vi "Set Mode (uSMC).vi"(8 "error in (no error)":errorcluster, 9 "Index":i32, 11 "Visa Array in":refnum<visa-resource-name>[](array[refnum])) -> (0 "error out":errorcluster, 3 "Visa Array out":refnum<visa-resource-name>[](array[refnum]))   [LabVIEW 2010, in "SignalWriterMH110203USBStepperMotor.lvclass"]
uses:
  SignalWriterMH110203USBStepperMotor.lvclass
  Mode Control (uSMC).ctl
  class_data.vi
panel:
  out "array buffer":u8[](array[numeric]) format="%b"
  out "element":T1={"Turn Buttons Off"=FALSE, "Reduce Current"=TRUE, "Power Off and Make a Whole Step"=TRUE, "Emergency Power Off"=FALSE, "Limit Switch 1 True State"=FALSE, "Limit Switch 2 True State"=FALSE, "Rotary Transducer TRUE State"=TRUE, "Swap Limit Switches"=TRUE, "Limit Switch 1 Operation Enabled"=TRUE, "Limit Switch 2 Operation Enabled"=TRUE, "Rotary Transducer Operation Enabled"=FALSE, "Rotary Transducer Operation Select"=TRUE, "Button 1 True State"=FALSE, "Button 2 True State"=FALSE, "Swap Buttons"=FALSE, "Reset Rotary Transducer Check Positions"=TRUE, "Output Syncronization Enabled"=FALSE, "Reset Output Sync Count"=FALSE, "Sync Operation"=FALSE, "Sync Count"=50, "Power"=TRUE, "Invert Sync Polarity"=FALSE, "Use Encoder"=FALSE, "Invert Encoder Direction"=FALSE, "Reset Encoder To 0"=FALSE, "Reset SM Enc Pos to Enc Pos"=FALSE}
  out "appended array":u8[](array[numeric]) format="%b"
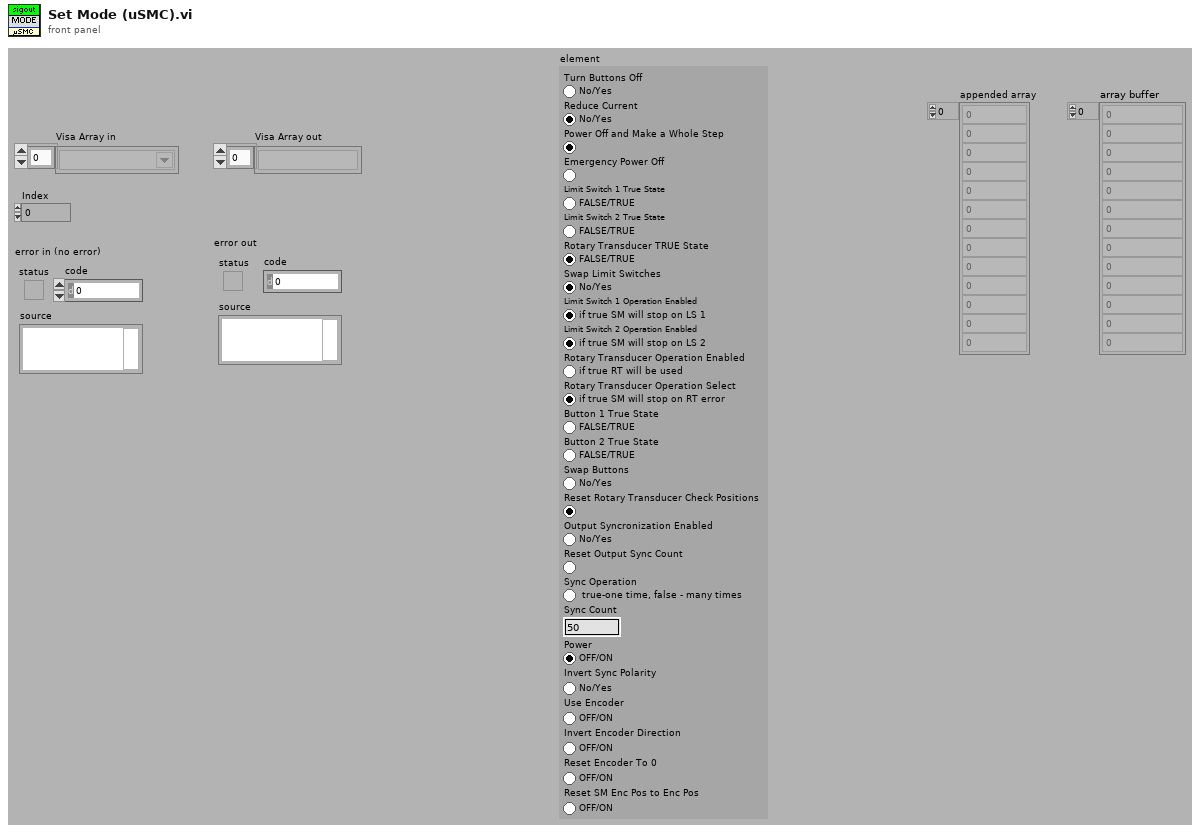
[diagram p1: front panel]
types:
  T1 = typedef "SignalWriterMH110203USBStepperMotor.lvclass/Mode Control (uSMC).ctl" = cluster{"Turn Buttons Off":bool, "Reduce Current":bool, "Power Off and Make a Whole Step":bool, "Emergency Power Off":bool, "Limit Switch 1 True State":bool, "Limit Switch 2 True State":bool, "Rotary Transducer TRUE State":bool, "Swap Limit Switches":bool, "Limit Switch 1 Operation Enabled":bool, "Limit Switch 2 Operation Enabled":bool, "Rotary Transducer Operation Enabled":bool, "Rotary Transducer Operation Select":bool, "Button 1 True State":bool, "Button 2 True State":bool, "Swap Buttons":bool, "Reset Rotary Transducer Check Positions":bool, "Output Syncronization Enabled":bool, "Reset Output Sync Count":bool, "Sync Operation":bool, "Sync Count":u32, "Power":bool, "Invert Sync Polarity":bool, "Use Encoder":bool, "Invert Encoder Direction":bool, "Reset Encoder To 0":bool, "Reset SM Enc Pos to Enc Pos":bool}
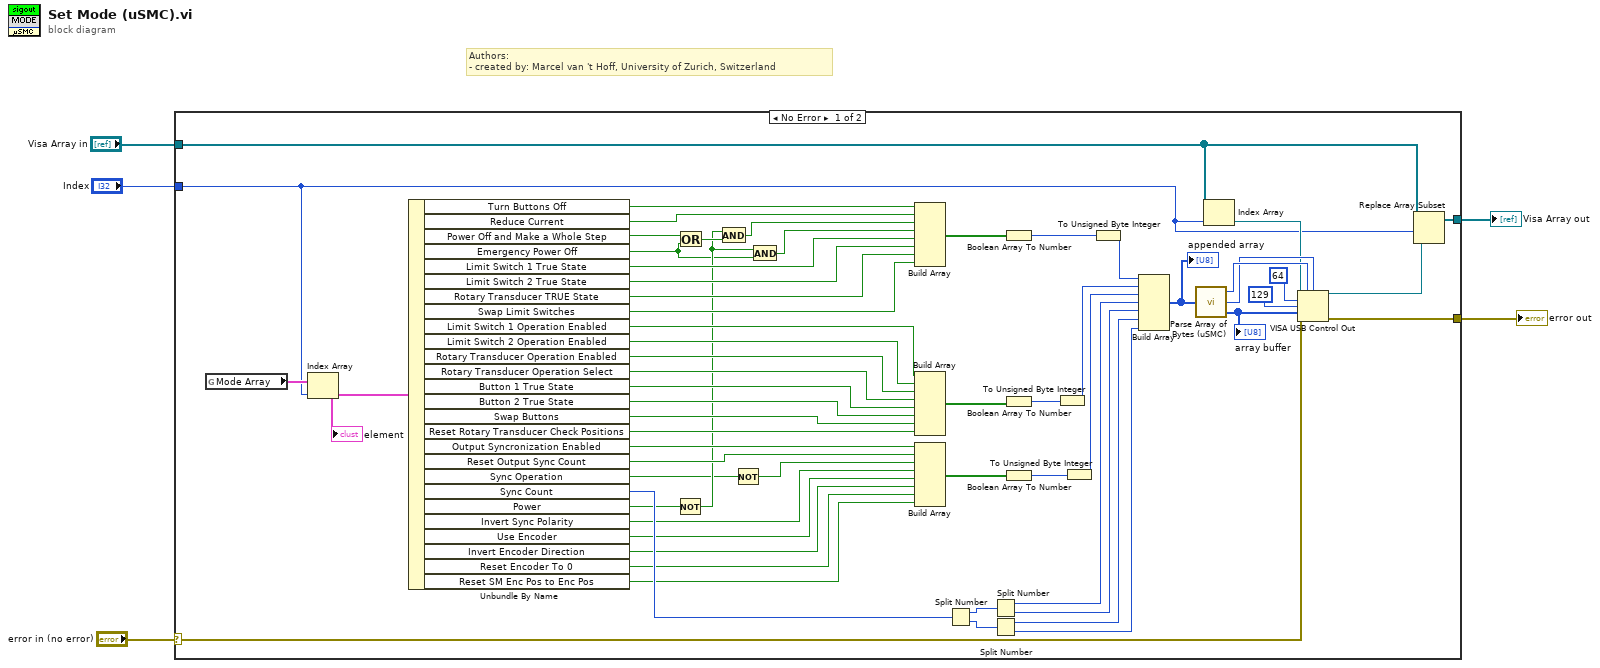
[diagram p0: block diagram]
diagram:
  # "Authors: \n- created by: Marcel van 't Hoff, University of Zurich, Switzerland"
  n1 = case shown="No Error" "error in (no error)" {
    selector: "error in (no error)" -> [w6 w68]
    tunnel: [w53 w68] -> w5
    tunnel: "Visa Array in" -> [w25 w67]
    tunnel: [w23 w67] -> w3
    tunnel: "Index" -> [w20 _]
    frame No Error {
      n2 = global read "class_data.vi" "Mode Array"() -> (w22:T1[])
      n3 = Index Array(array=w22, index=w20) -> (element=w21:T1)
      "element" <- w21
      n4 = Unbundle By Name(w21) -> ("Turn Buttons Off"=w45:bool, "Reduce Current"=w44:bool, "Power Off and Make a Whole Step"=w43:bool, "Emergency Power Off"=w15:bool, "Limit Switch 1 True State"=w42:bool, "Limit Switch 2 True State"=w41:bool, "Rotary Transducer TRUE State"=w40:bool, "Swap Limit Switches"=w39:bool, "Limit Switch 1 Operation Enabled"=w37:bool, "Limit Switch 2 Operation Enabled"=w36:bool, "Rotary Transducer Operation Enabled"=w35:bool, "Rotary Transducer Operation Select"=w34:bool, "Button 1 True State"=w33:bool, "Button 2 True State"=w32:bool, "Swap Buttons"=w31:bool, "Reset Rotary Transducer Check Positions"=w30:bool, "Output Syncronization Enabled"=w29:bool, "Reset Output Sync Count"=w28:bool, "Sync Operation"=w14:bool, "Sync Count"=w27:u32, "Power"=w11:bool, "Invert Sync Polarity"=w12:bool, "Use Encoder"=w10:bool, "Invert Encoder Direction"=w9:bool, "Reset Encoder To 0"=w8:bool, "Reset SM Enc Pos to Enc Pos"=w7:bool)
      n5 = Not(x=w11) -> (.not. x?=w16:bool)
      n6 = Or(x=w43, y=w15) -> (x .or. y?=w19:bool)
      n7 = And(x=w16, y=w19) -> (x .and. y?=w18:bool)
      n8 = Not(x=w14) -> (.not. x?=w13:bool)
      n9 = And(x=w16, y=w15) -> (x .and. y?=w17:bool)
      n10 = Build Array(w45, w44, w18, w17, w42, w41, w40, w39) -> (w64:bool[])
      n11 = Build Array(w37, w36, w35, w34, w33, w32, w31, w30) -> (w38:bool[])
      n12 = Build Array(w29, w28, w13, w12, w10, w9, w8, w7) -> (w60:bool[])
      n13 = Split Number(x=w27) -> (hi(x)=w66:u16, lo(x)=w65:u16)
      n14 = Split Number(x=w66) -> (hi(x)=w46:u8, lo(x)=w59:u8)
      n15 = Split Number(x=w65) -> (hi(x)=w58:u8, lo(x)=w57:u8)
      n16 = Boolean Array To Number(Boolean array=w64) -> (number=w63:u32)
      n17 = Boolean Array To Number(Boolean array=w38) -> (number=w62:u32)
      n18 = Boolean Array To Number(Boolean array=w60) -> (number=w61:u32)
      n19 = To Unsigned Byte Integer(number=w62) -> (unsigned 8bit integer=w48:u8)
      n20 = To Unsigned Byte Integer(number=w61) -> (unsigned 8bit integer=w47:u8)
      n21 = To Unsigned Byte Integer(number=w63) -> (unsigned 8bit integer=w49:u8)
      n22 = Build Array(w49, w48, w47, w46, w59, w58, w57) -> (w56:u8[])
      "appended array" <- w56
      n23 = call "Parse Array of Bytes (uSMC).vi"("byte array"=w56) -> ("first 2 bytes"=w51:u16, "second 2 bytes"=w50:u16, "array buffer"=w52:u8[])
      "array buffer" <- w52
      n24 = Index Array(array=w25, index=w20) -> (element=w26:refnum<visa-resource-name>)
      n25 = VISA USB Control Out(0:w26, 1:w51, 2:w50, 5:i16 64 ("request type"), 7:i16 129 ("request type"), 9:w52, 11:w6) -> (4:w24:refnum<visa-resource-name>, 15:w53:errorcluster)
      n26 = Replace Array Subset(array=w25, new element=w24, index=w20) -> (w23:refnum<visa-resource-name>[])
    }
    frame Error {
    }
  }
  "error out" <- w5
  "Visa Array out" <- w3
